vi "AC_Source_VISA.vi"(4 "error_in":errorcluster, 5 "Parameter":T1, 6 "Mode":T2(ring)=enum."TurnOn", 7 "VISA_in":refnum<visa-resource-name>) -> (0 "error_out":errorcluster, 1 "Parameter 2":T1, 3 "VISA_out":refnum<visa-resource-name>)   [LabVIEW 2019]
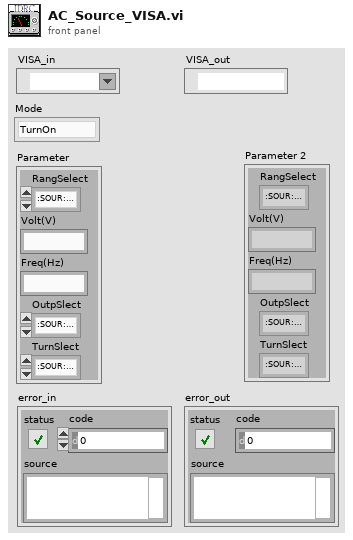
[diagram p1: front panel]
types:
  T1 = cluster{"RangSelect":enum16{":SOUR:RANG LOW;", ":SOUR:RANG HIGH;", ":SOUR:RANG AUTO;"}, "Volt(V)":string, "Freq(Hz)":string, "OutpSlect":enum16{":SOUR:TURN OFF;", ":SOUR:TURN ON;"}, "TurnSlect":enum16{":SOUR:TURN OFF;", ":SOUR:TURN ON;"}}
  T2 = enum16{"SetRange", "SetVoltage", "SetFreq", "OUTP", "TurnOn"}
  T3 = enum16{":SOUR:RANG LOW;", ":SOUR:RANG HIGH;", ":SOUR:RANG AUTO;"}
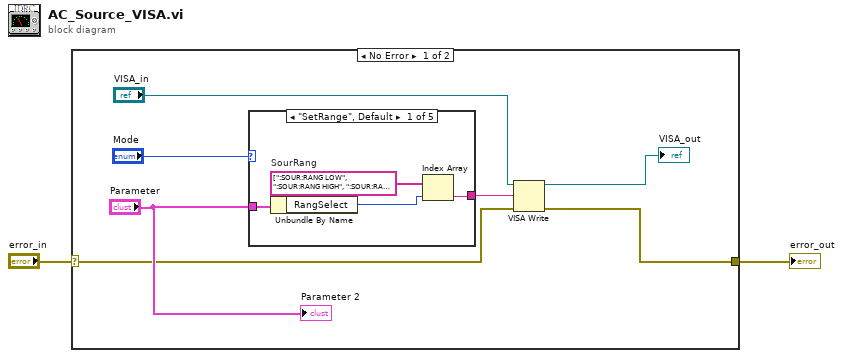
[diagram p0: block diagram]
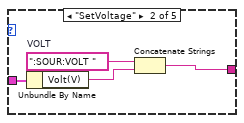
[diagram p2: hidden frame]
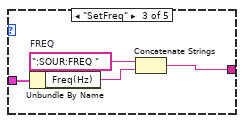
[diagram p3: hidden frame]
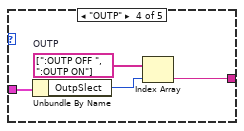
[diagram p4: hidden frame]
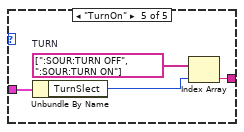
[diagram p5: hidden frame]
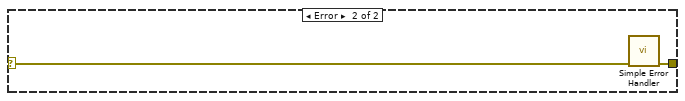
[diagram p6: hidden frame]
diagram:
  n1 = case shown="No Error" "error_in" {
    selector: "error_in" -> [w6 w31]
    tunnel: [w4 w30] -> w1
    frame No Error {
      n2 = case shown="\"SetRange\", Default" "Mode" {
        tunnel: "Parameter" -> [w12 w16 w20 w24 w28]
        tunnel: [w10 w14 w18 w23 w26] -> w7
        frame "SetRange", Default {
          w13 = string[] [":SOUR:RANG LOW", ":SOUR:RANG HIGH", ":SOUR:RANG AUTO;"]  # SourRang
          n3 = Unbundle By Name(w12) -> ("RangSelect"=w11:T3)
          n4 = Index Array(array=w13, index=w11) -> (element=w10:string)
        }
        frame "SetVoltage" {
          w17 = ":SOUR:VOLT "  # VOLT
          n5 = Unbundle By Name(w16) -> ("Volt(V)"=w15:string)
          n6 = Concatenate Strings(w17, w15) -> (w14:string)
        }
        frame "SetFreq" {
          w21 = ":SOUR:FREQ "  # FREQ
          n7 = Unbundle By Name(w20) -> ("Freq(Hz)"=w19:string)
          n8 = Concatenate Strings(w21, w19) -> (w18:string)
        }
        frame "OUTP" {
          w25 = string[] [":OUTP OFF ", ":OUTP ON"]  # OUTP
          n9 = Unbundle By Name(w24) -> ("OutpSlect"=w22:enum16{":SOUR:TURN OFF;", ":SOUR:TURN ON;"})
          n10 = Index Array(array=w25, index=w22) -> (element=w23:string)
        }
        frame "TurnOn" {
          w29 = string[] [":SOUR:TURN OFF", ":SOUR:TURN ON"]  # TURN
          n11 = Unbundle By Name(w28) -> ("TurnSlect"=w27:enum16{":SOUR:TURN OFF;", ":SOUR:TURN ON;"})
          n12 = Index Array(array=w29, index=w27) -> (element=w26:string)
        }
      }
      n13 = VISA Write(VISA resource name="VISA_in", write buffer=w7, error in (no error)=w6) -> (VISA resource name out=→"VISA_out":refnum<visa-resource-name>, error out=w4:errorcluster)  [unwired: 1 out]
      "Parameter 2" <- "Parameter"
    }
    frame Error {
      n14 = call <vilib>:"Simple Error Handler.vi"("error in (no error)"=w31) -> ("error out"=w30:errorcluster)  [unwired: 4 in, 4 out]
    }
  }
  "error_out" <- w1
